vi "SortControlsAndIndicators.vi"(8 "error in":errorcluster, 10 "Controls[]":refnum<vi>[](array[refnum]), 11 "LVClassLibrary Refnum":refnum<vi>) -> (0 "error out":errorcluster, 1 "Controls":refnum<vi>[](array[refnum]), 2 "Indicators":refnum<vi>[](array[refnum]), 3 "Library Refnum out":refnum<vi>)   [LabVIEW 2014, in "ClassRenamer.lvclass"]
uses:
  ClassRenamer.lvclass
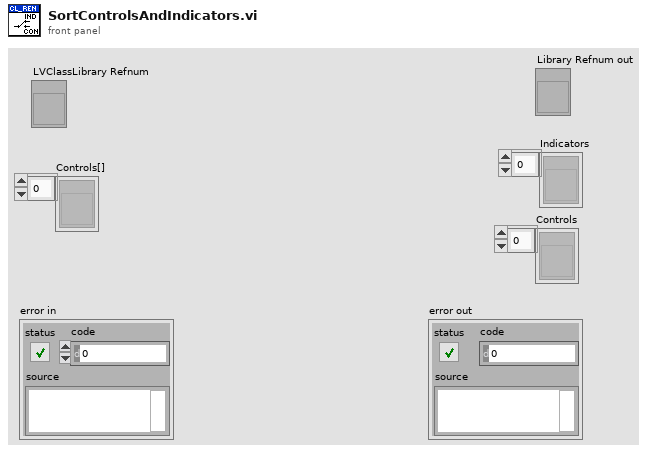
[diagram p1: front panel]
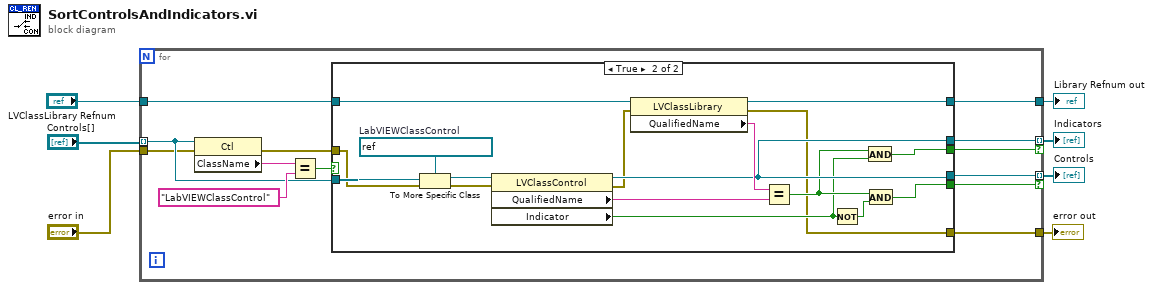
[diagram p0: block diagram]
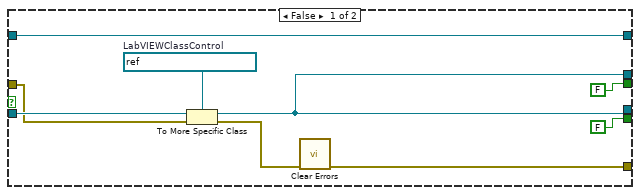
[diagram p2: hidden frame]
diagram:
  n1 = for {
    tunnel: "Controls[]" -> [w17] mode=indexing
    tunnel: "LVClassLibrary Refnum" -> [w16]
    tunnel: [w15] -> w6 mode=indexing if=w13
    tunnel: [w14] -> w7 mode=indexing if=w12
    tunnel: "error in" -> [w11]
    tunnel: [w9] -> w2
    tunnel: [w8] -> w1
    n2 = property class="Ctl"(reference=w17, error in=w11) -> (error out=w10:errorcluster, "ClassName"=w19:string)  [unwired: 1 out]
    n3 = Equal?(x=w19, y="LabVIEWClassControl" ("Terminal.ClassName")) -> (x = y?=w18:bool)
    n4 = case shown="True" w18 {
      tunnel: w17 -> [w26 w46]
      tunnel: w16 -> [w23 w43]
      tunnel: [w25 w39] -> w15
      tunnel: [FALSE w40] -> w13
      tunnel: [w25 w39] -> w14
      tunnel: [FALSE w35] -> w12
      tunnel: w10 -> [w22 w34]
      tunnel: [w23 w31] -> w9
      tunnel: [w21 w30] -> w8
      frame False {
        w27 = refnum<vi> refnum  # LabVIEWClassControl
        n5 = To More Specific Class(target class=w27, reference=w26, error in=w22) -> (specific class reference=w25:refnum<vi>, error out=w24:errorcluster)
        n6 = call <vilib>:"Clear Errors.vi"("error in (no error)"=w24) -> ("error out"=w21:errorcluster)  [unwired: 5 in, 1 out]
      }
      frame True {
        w45 = refnum<vi> refnum  # LabVIEWClassControl
        n7 = To More Specific Class(target class=w45, reference=w46, error in=w34) -> (specific class reference=w44:refnum<vi>, error out=w33:errorcluster)
        n8 = property class="LVClassControl"(reference=w44, error in=w33) -> (reference out=w39:refnum<vi>, error out=w32:errorcluster, "QualifiedName"=w41:string, "Indicator"=w37:bool)
        n9 = property class="LVClassLibrary"(reference=w43, error in=w32) -> (reference out=w31:refnum<vi>, error out=w30:errorcluster, "QualifiedName"=w42:string)
        n10 = Equal?(x=w42, y=w41) -> (x = y?=w38:bool)
        n11 = Not(x=w37) -> (.not. x?=w36:bool)
        n12 = And(x=w38, y=w37) -> (x .and. y?=w40:bool)
        n13 = And(x=w38, y=w36) -> (x .and. y?=w35:bool)
      }
    }
  }
  "Controls" <- w7
  "Indicators" <- w6
  "Library Refnum out" <- w2
  "error out" <- w1
